vi "ChangeFilter.vi"(8 "error in (no error)":errorcluster) -> ()   [LabVIEW 2012]
doc: "PowerDemo.vi\nThe Demo enables power measurement and display results.\nVersion 1.00\nLast Updated 16 Mars 2005\n\nDemo Program Steps:\n \n1) The vi executes InitCom.vi to open the communication session.\nThe default is RS232,Port2,9600 bps and Address 10 for USB.\n\nYou have to select USB or RS232 Protocol and\nupdate these values for any change.\n\n2) The vi executes ConfMeasure.vi to Send \"FP\" (Force Power) to Device and \"SI\" (Send unIts) to receive the units\n\n3) The vi executes a loop of SendPower.vi to get measurements.\nWhen no Overrange value the vi add value to array for update\nstatistics values.\n\nIn case of Error:\nError Out contains the Error Number and the vi's name where the error occured.\n\nVISA Error Codes -10738077360 to -1073807231\nOphir Error Codes -1300 to 1340"
panel:
  out "Frame Output":string
  out "Ophir Board":string
  out "Debug Index":i32
  out "error out":errorcluster
  out "dup Visa Session":refnum<visa-resource-name>
  out "Device Response":string="\r\n"
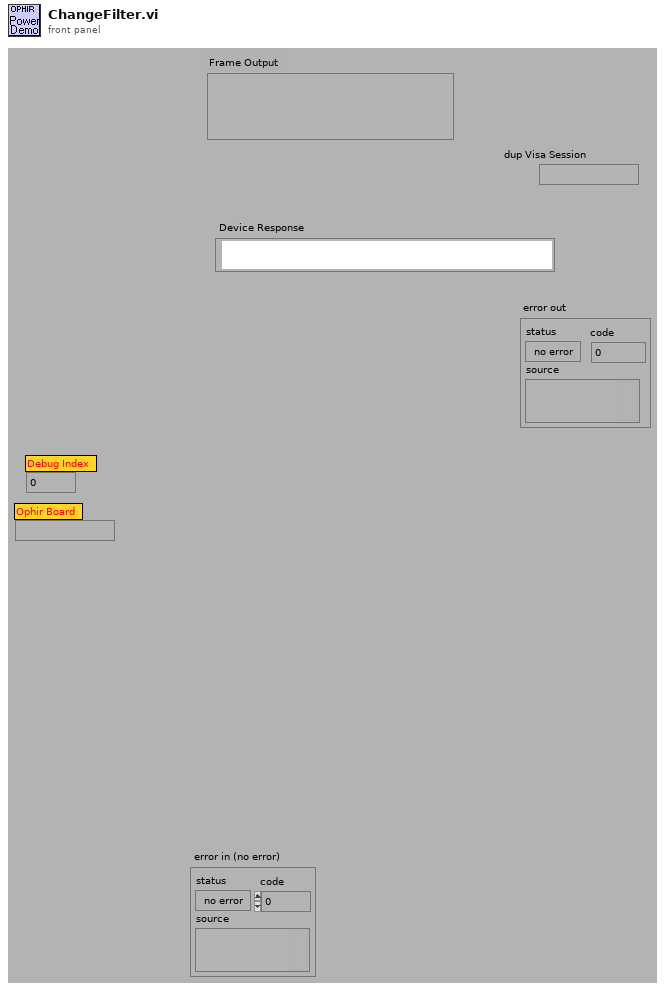
[diagram p1: front panel]
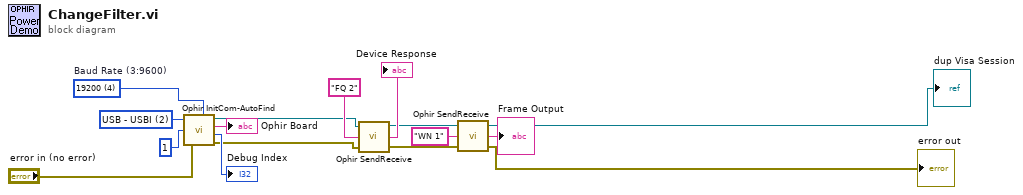
[diagram p0: block diagram]
diagram:
  w12 = i16 4 items=["300", "1200", "4800", "9600", "19200", "38400"]  # Baud Rate (3:9600)
  w10 = i16 2 items=["USB - Nova2", "USB - Vega", "USB - USBI", "RS232", "GPIB"] ("communication")
  n1 = call "Ophir InitCom-AutoFind.vi"("Baud Rate (3:9600)"=w12, "communication"=w10, "Port Number (default 2)"=i16 1, "error in (no error)"="error in (no error)") -> ("Dup Visa Session"=w9:refnum<visa-resource-name>, "Ophir Board"=→"Ophir Board":string, "Debug Index"=→"Debug Index":i32, "error out"=w8:errorcluster)
  n2 = call "Ophir SendReceive.vi"("error in (no error)"=w8, "Command"="FQ 2", "Visa Session"=w9) -> ("error out"=w5:errorcluster, "Frame Output"=→"Device Response":string, "dup Visa Session"=w6:refnum<visa-resource-name>)
  n3 = call "Ophir SendReceive.vi"("error in (no error)"=w5, "Command"="WN 1", "Visa Session"=w6) -> ("error out"=→"error out":errorcluster, "Frame Output"=→"Frame Output":string, "dup Visa Session"=→"dup Visa Session":refnum<visa-resource-name>)
